vi "Read Exporter names.vi"(11 "UIManager in":refnum<class "UIManager.lvclass">) -> (1 "Exporter names":string[](array[string]), 3 "UIManager out":refnum<class "UIManager.lvclass">)   [LabVIEW 2020, in "DependencyInspector.lvlib" / "UIManager.lvclass"]
uses:
  UIManager.lvclass
  UIManager.lvclass/UIManager.ctl
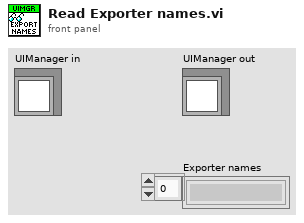
[diagram p1: front panel]
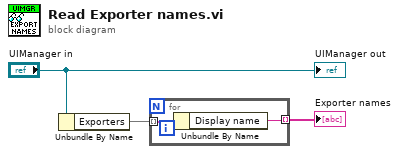
[diagram p0: block diagram]
diagram:
  n1 = Unbundle By Name("UIManager in") -> ("Exporters"=w1:map{string, refnum<class "IExporter.lvclass">})
  n2 = for {
    tunnel: w1 -> [w5] mode=indexing
    tunnel: [w4] -> w2 mode=indexing
    n3 = Unbundle By Name(w5) -> ("Display name"=w4:string)
  }
  "Exporter names" <- w2
  "UIManager out" <- "UIManager in"
